vi "Avocent_power_status.vi"(8 "error in":errorcluster, 11 "Power Status (raw string)":string="HTTP/1.1 200 OK\r\nDate: Wed, 05 Apr 2006 02:53:05 GMT\r\nExpires: Wed, 05 Apr 2006 02:52:05 GMT\r\nCache-control: private\r\nContent-type: text/html\r\n\r\n<table style=\"visibility: hidden\">\r\n\t<input  id =\"Z1\" name=111111111111111111111111,5,0,1, type=\"text\" style=\"visibility: hidden\">\r\n</table>\r\n") -> (0 "error out":errorcluster, 3 "Power status (boolean)":bool[](array[boolean])=[TRUE, TRUE, TRUE, TRUE, TRUE, TRUE, TRUE, TRUE, TRUE, TRUE, TRUE, TRUE, TRUE, TRUE, TRUE, TRUE, FALSE, FALSE, FALSE, FALSE, FALSE, FALSE, FALSE, FALSE, FALSE, FALSE, FALSE, FALSE, FALSE, FALSE, FALSE, FALSE] caption="Power indicator")   [LabVIEW 2013]
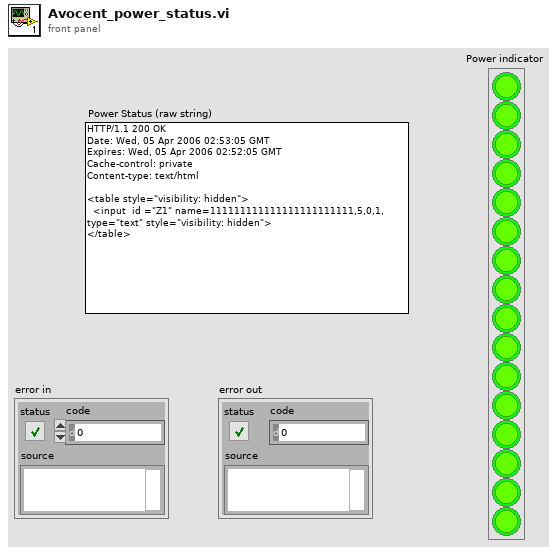
[diagram p1: front panel]
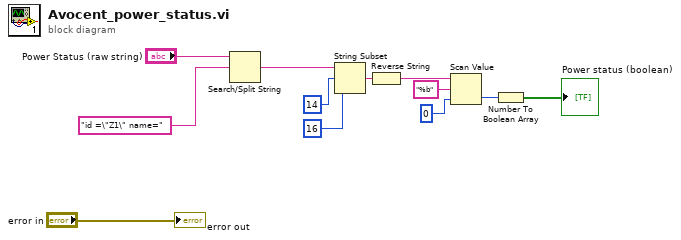
[diagram p0: block diagram]
diagram:
  n1 = Search/Split String(string="Power Status (raw string)", search string/char (-)="id =\"Z1\" name=") -> (match + rest of string=w11:string)  [unwired: 1 in, 2 out]
  n2 = String Subset(string=w11, offset (0)=14, length (rest)=16) -> (substring=w6:string)
  n3 = Reverse String(1:w6) -> (0:w4:string)
  n4 = Scan Value(string=w4, format string="%b", default (0 dbl)=u32 0 ("number")) -> (value=w5:u32)  [unwired: 1 out]
  n5 = Number To Boolean Array(number=w5) -> (Boolean array=→"Power status (boolean)":bool[])
  "error out" <- "error in"
